vi "broadcast_handshake.vi"(8 "error in (no error)":errorcluster, 11 "RemoteAnalysisToolKit in":refnum<class "RemoteAnalysisToolKit.lvclass">) -> (0 "error out":errorcluster, 3 "RemoteAnalysisToolKit out":refnum<class "RemoteAnalysisToolKit.lvclass">)   [LabVIEW 2010, in "RemoteAnalysisToolKit.lvclass"]
uses:
  RemoteAnalysisToolKit.lvclass
  RemoteAnalysisToolKit.lvclass/RemoteAnalysisToolKit.ctl
  <vilib>/Utility/tcp.llb/UDP Multicast Open.vi
  <vilib>/Utility/tcp.llb/UDP Multicast Read-Write Open.vi
panel:
  out "data out":string
  in  "stop":bool
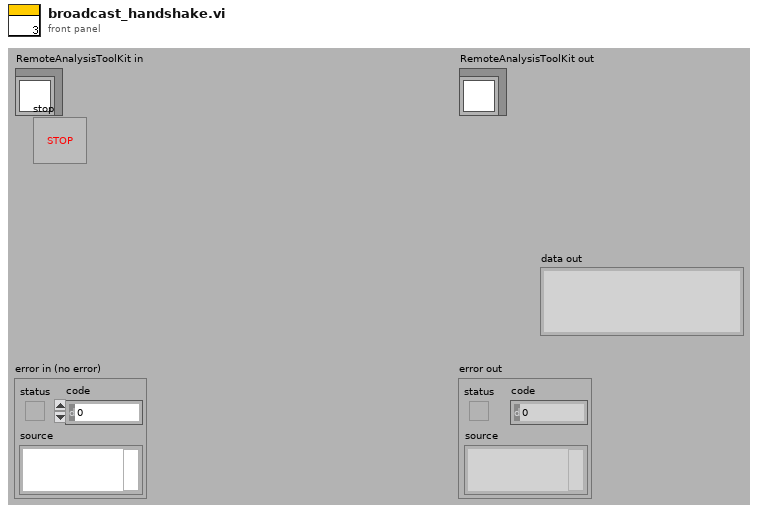
[diagram p1: front panel]
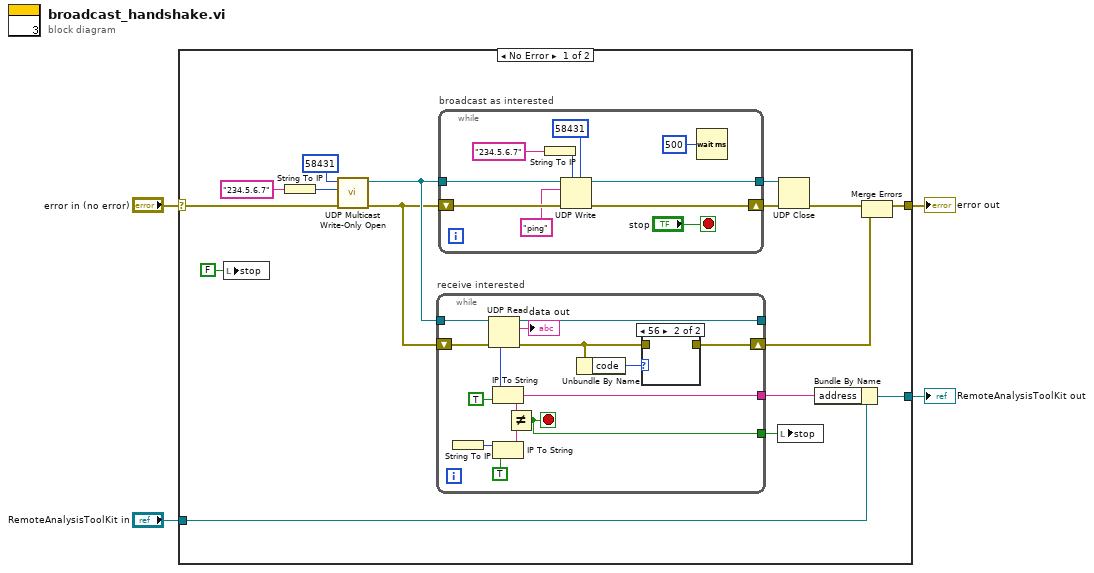
[diagram p0: block diagram]
diagram:
  n1 = case shown="No Error" "error in (no error)" {
    selector: "error in (no error)" -> [w9 w47]
    tunnel: [w8 w47] -> w3
    tunnel: [w6 w46] -> w1
    tunnel: "RemoteAnalysisToolKit in" -> [w7 w46]
    frame No Error {
      n2 = local write "stop"(FALSE ("stop")) -> ()
      n3 = String To IP(1:"234.5.6.7" ("Multicast Address")) -> (0:w14:u32)
      n4 = call-poly "UDP Multicast Write-Only Open.vi"("error in (no error)"=w9, "multicast addr"=w14, "port"=u16 58431) -> ("error out"=w16:errorcluster, "connection ID"=w17:refnum<k16>)  [unwired: 6 in, 1 out]
      n5 = while "receive interested" {
        tunnel: [w34] -> _
        tunnel: w17 -> [w32]
        shift-right: [w28] -> w11
        shift-left: w16 -> [w31]
        tunnel: [w22] -> w5
        tunnel: [w21] -> w13
        stop <- w21 stop-if-true
        n6 = String To IP() -> (0:w25:u32)  [unwired: 1 in]
        n7 = UDP Read(connection ID=w32, 8:w31) -> (data out=→"data out":string, error out=w29:errorcluster, 3:w34:refnum<k16>, 6:w26:u32)  [unwired: 1 in, 2 out]
        n8 = IP To String(1:TRUE ("dot notation? (F)"), 2:w26) -> (0:w22:string)
        n9 = IP To String(1:TRUE ("dot notation? (F)"), 2:w25) -> (0:w23:string)
        n10 = Not Equal?(x=w22, y=w23) -> (x != y?=w21:bool)
        n11 = Unbundle By Name(w29) -> ("code"=w30:i32)
        n12 = case shown="56" w30 {
          tunnel: w29 -> [w35 _]
          tunnel: [w35 _] -> w28
          frame Default {
          }
          frame 56 {
          }
        }
      }
      n13 = while "broadcast as interested" {
        tunnel: [w41] -> w19
        tunnel: w17 -> [w37]
        shift-right: [w40] -> w20
        shift-left: w16 -> [w38]
        stop <- "stop" stop-if-true
        n14 = String To IP(1:"234.5.6.7" ("Multicast Address")) -> (0:w43:u32)
        n15 = UDP Write(address=w43, port or service name=u16 58431 ("Send to Port"), connection ID=w37, data in="ping", 8:w38) -> (error out=w40:errorcluster, 3:w41:refnum<k16>)  [unwired: 1 in]
        n16 = Wait (ms)(milliseconds to wait=u32 500) -> ()  [unwired: 1 out]
      }
      n17 = local write "stop"(w13) -> ()
      n18 = UDP Close(connection ID=w19, 8:w20) -> (error out=w12:errorcluster)  [unwired: 1 out]
      n19 = Bundle By Name(cluster=w7, "address"=w5) -> (w6:refnum<class "RemoteAnalysisToolKit.lvclass">)
      n20 = Merge Errors(w12, w11) -> (w8:errorcluster)
    }
    frame Error {
    }
  }
  "error out" <- w3
  "RemoteAnalysisToolKit out" <- w1
